vi "Test Get Table Column Cell Value.vi"(11 "Test Case In":refnum<class "Test Open Xml.lvclass">) -> (0 "error out":errorcluster, 3 "Test Case Out":refnum<class "Test Open Xml.lvclass">)   [LabVIEW 2020, in "Test Open Xml.lvclass"]
uses:
  Test Open Xml.lvclass
  C:/Program Files/National Instruments/LabVIEW 2025/vi.lib/Astemes/LUnit/Test Case.lvclass
  <vilib>/Astemes/LUnit/Test Case.lvclass/Test Case.ctl
  0a0d70f3-36fe-46ba-8b3e-e6c07e708d9f.vi
  <vilib>/Astemes/LUnit/Core/LUnit Test Case/Private/Append Pass Result.vi
  <vilib>/Astemes/LUnit/Core/LUnit Test Case/Private/Append Fail Result.vi
  0a0d70f3-36fe-46ba-8b3e-e6c07e708d9f.vi/9c5d11cd-9439-4240-a1ee-d9baace9c924.vi
  <vilib>/Astemes/LUnit/Core/LUnit Test Case/Private/Run In UI.vi
  <vilib>/Utility/error.llb/Clear Errors.vi
  Source/Open Xml.lvlib
panel:
  out "appended array":variant[][](array[variant])
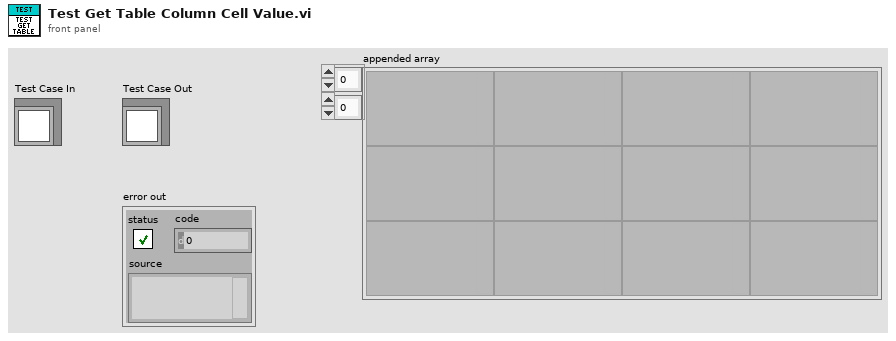
[diagram p1: front panel]
types:
  T1 = cluster{"Sheet Name":string, "Name":string, "Display Name":string, "Range":string}
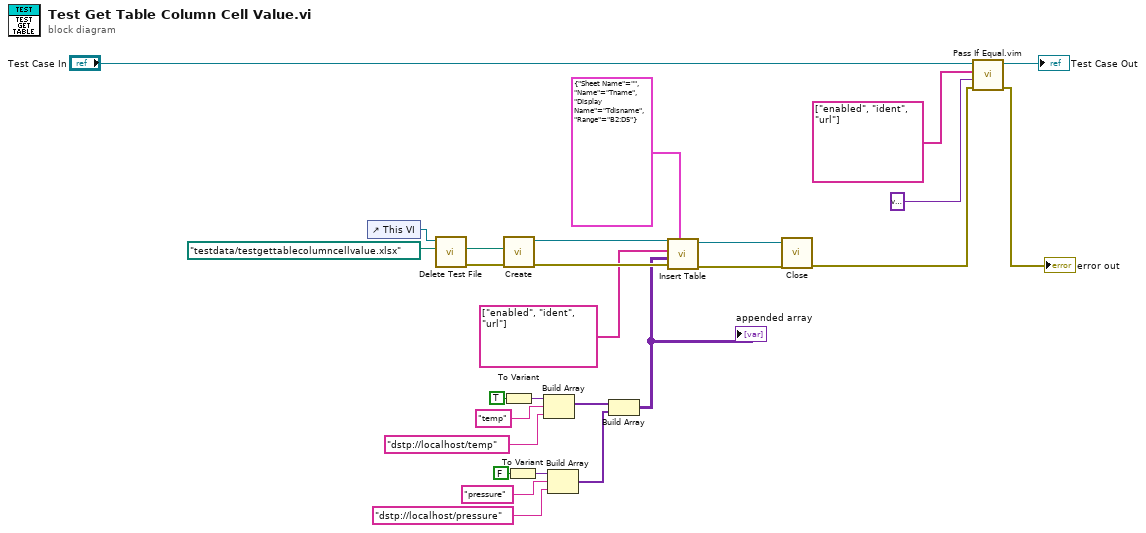
[diagram p0: block diagram]
diagram:
  n1 = control-ref of="This VI"() -> (w17:refnum<vi>)
  n2 = call "Delete Test File.vi"("name or relative path"=path "testdata/testgettablecolumncellvalue.xlsx", "VI in"=w17) -> ("error out"=w18:errorcluster, "deleted path"=w19:path)  [unwired: 8 in]
  n3 = call "Create.vi"("error in"=w18, "Path"=w19) -> ("error out"=w14:errorcluster, "SpreadsheetDoc"=w15:refnum<k24>)  [unwired: 8 in]
  n4 = To Variant(anything=TRUE) -> (Variant=w11:variant)
  n5 = To Variant(anything=FALSE) -> (Variant=w6:variant)
  n6 = Build Array(w11, "temp", "dstp://localhost/temp") -> (w4:variant[])
  n7 = Build Array(w6, "pressure", "dstp://localhost/pressure") -> (w3:variant[])
  n8 = Build Array(w4, w3) -> (w1:variant[][])
  "appended array" <- w1
  n9 = call "Insert Table.vi"("Location"=T1 {"Sheet Name"="", "Name"="Tname", "Display Name"="Tdisname", "Range"="B2:D5"}, "error in"=w14, "Cell Values"=w1, "Header Names"=string[] ["enabled", "ident", "url"], "SpreadsheetDoc in"=w15) -> ("error out"=w22:errorcluster, "SpreadsheetDoc out"=w21:refnum<k24>)  [unwired: 4 in, 1 out]
  n10 = call "Close.vi"("error in"=w22, "SpreadsheetDoc"=w21) -> ("error out"=w24:errorcluster)  [unwired: 9 in]
  n11 = call "Pass If Equal.vim"("error in (no error)"=w24, "Actual"=variant, "Expected"=string[] ["enabled", "ident", "url"] ("Headers"), "LUnit Test Case In"="Test Case In") -> ("error out"=→"error out":errorcluster, "LUnit Test Case Out"=→"Test Case Out":refnum<class "Test Open Xml.lvclass">)  [unwired: 6 in]
